vi "Post-Post-Build Action.vi"() -> ()   [LabVIEW 2020]
uses:
  <vilib>/JKI/VIPM API/command-line/support/Version Info Cluster_vipm_api.ctl
  <vilib>/Utility/miscctls.llb/LVMapReplaceAction.ctl
  <vilib>/Utility/traverseref.llb/TRef TravTarget.ctl
  cd8b867b-32d4-4915-be8a-6b797f053483.vi
  2e8c776f-19e2-48a1-b577-1ff0846f967f.vi
  383cdb5e-1483-4389-8633-9a82e05b406f.vi
  da8bf82a-4c59-4cf2-9509-83ebec40744a.vi
  <vilib>/Utility/traverseref.llb/VI Scripting - Traverse.lvlib
  <vilib>/JKI/VIPM API/VIPM API_vipm_api.lvlib
panel:
  out "File":path
  out "Action":string
  in  "Folder Path":path caption="Folder Path (Empty: Source Distrubution Built Folder)"
  # "Run this after the source distribution build and outside of the main project to avoid crashes/cross linking to VI.lib"
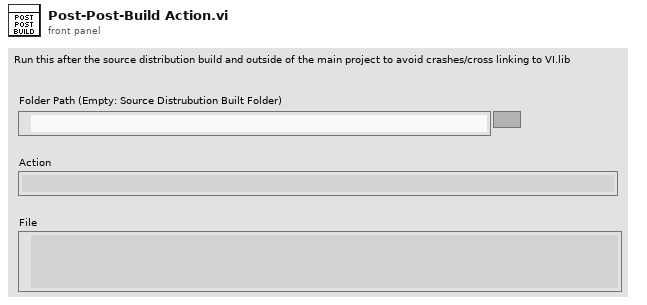
[diagram p1: front panel]
types:
  T1 = typedef "VIPM API_vipm_api.lvlib/Version Info Cluster_vipm_api.ctl" = cluster{"major":u32, "minor":u32, "patch":u32, "build":u32}
  T2 = cluster{"Vims":map{path, path[]}, "Src Files":path[]}
  T3 = cluster{"Source Distribution":path, "vi.lib Binary Source Dir":path, "Binary Source Dir":path}
  T4 = enum16{"Compute Paths", "Scan for .vims", "Inline .vims", "Delete .vims from Libs & Disk", "Rewildcard Paths before zip", "Zip", "Copy Binaries to vi.lib"}
  T5 = enum16{"Compute Paths", "Scan for .vims", "Inline .vims", "Delete .vims from Libs & Disk", "Rewildcard Paths before zip", "Zip", "Copy Binaries to vi.lib"}[]
  T6 = typedef "LVMapReplaceAction.ctl" = enum32{"Modify Entry only if found", "Add or Modify Entry", "Delete Entry"}
  T7 = typedef "TRef TravTarget.ctl" = enum16{"FP", "BD", "Other"}
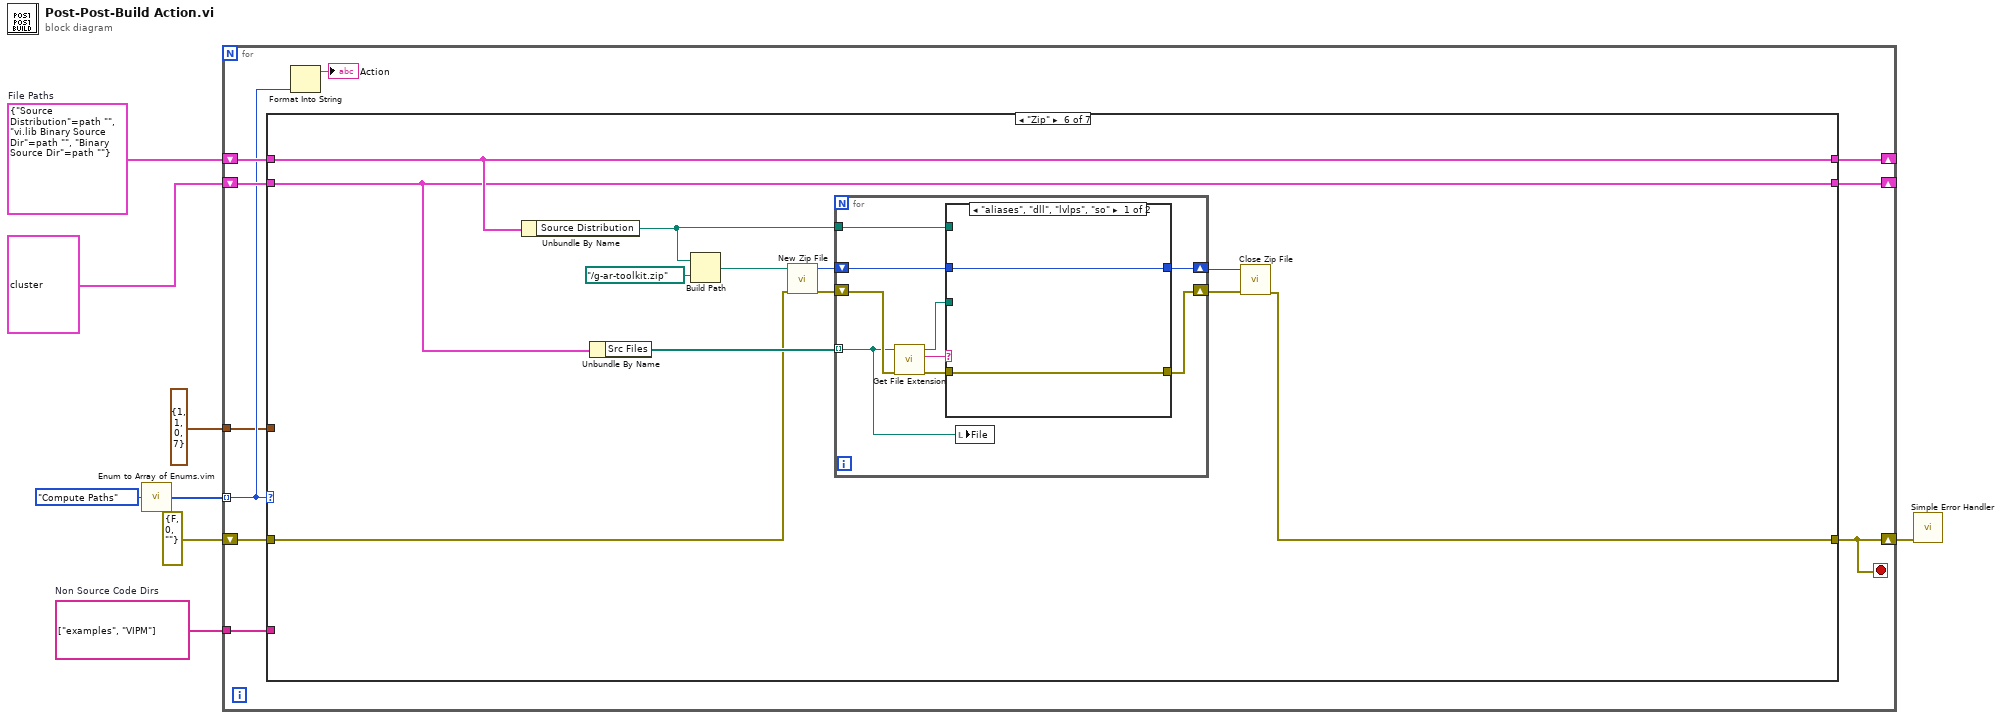
[diagram p0: block diagram]
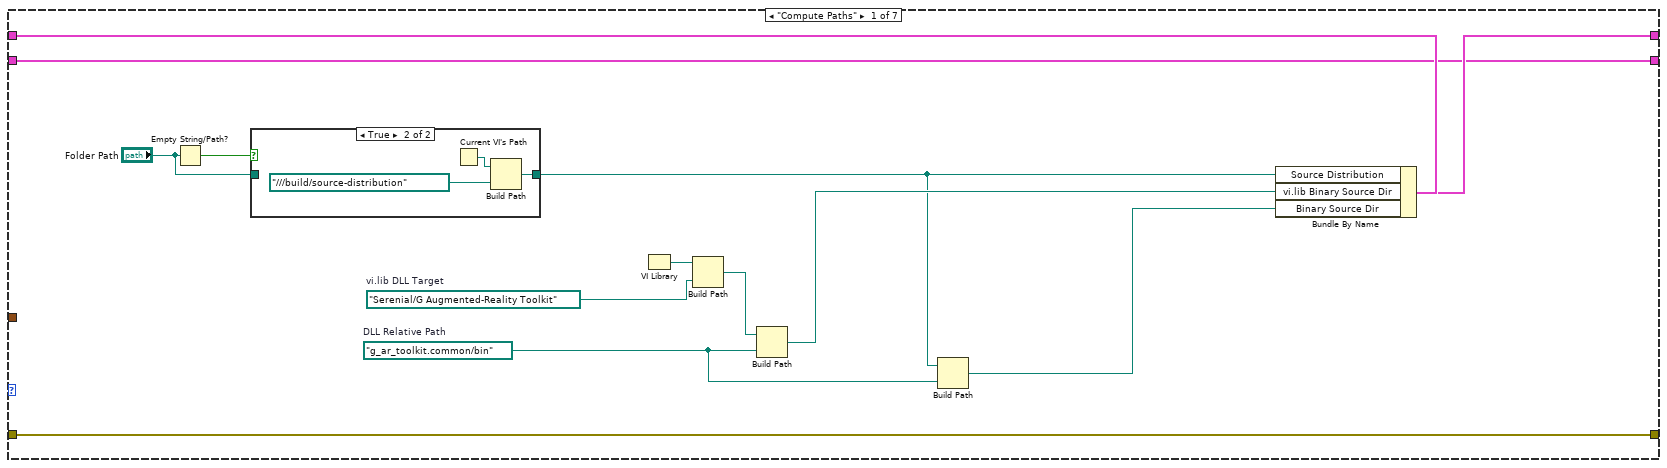
[diagram p2: hidden frame]
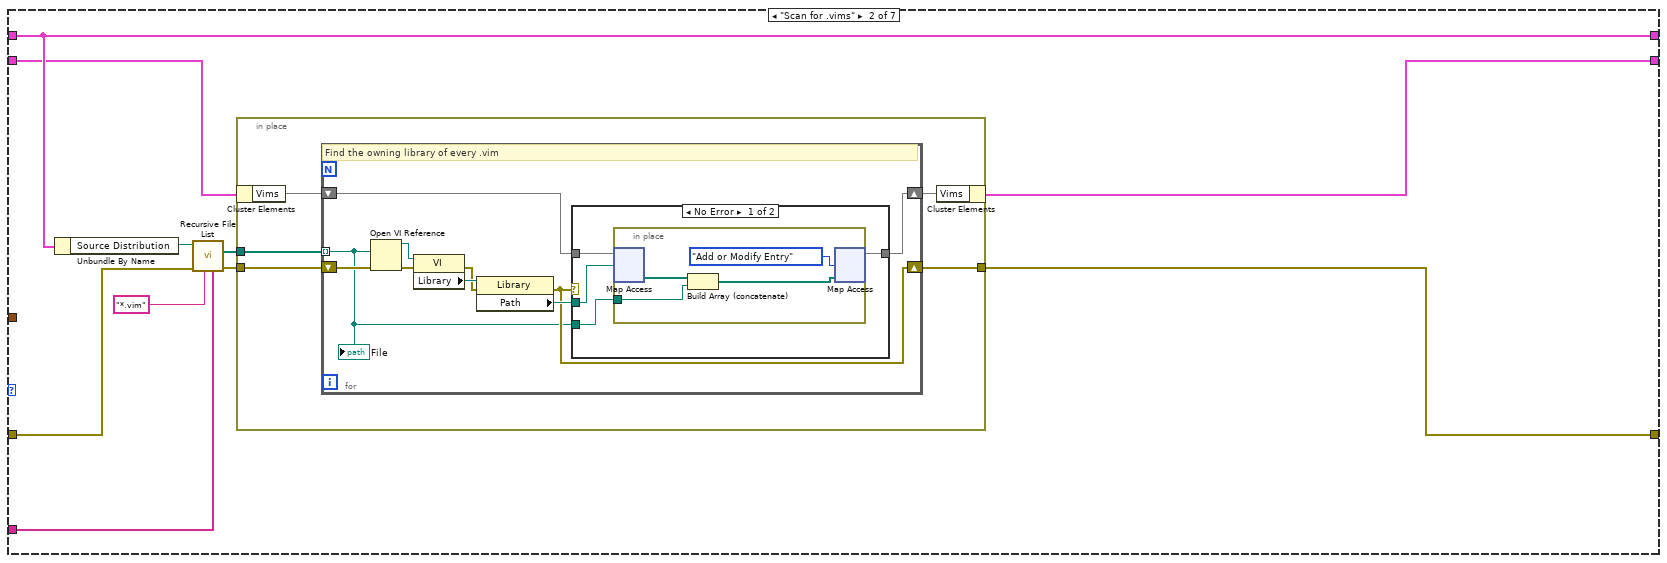
[diagram p4: hidden frame]
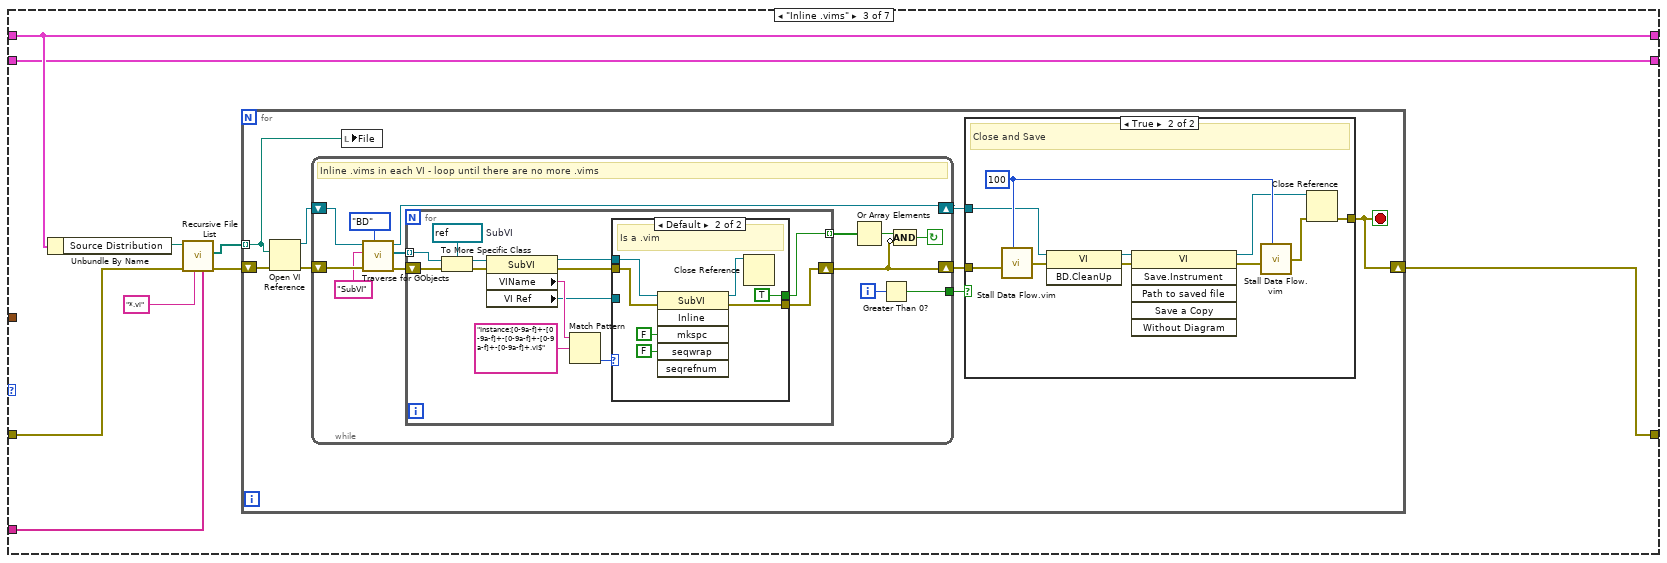
[diagram p6: hidden frame]
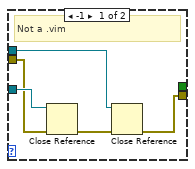
[diagram p7: hidden frame]
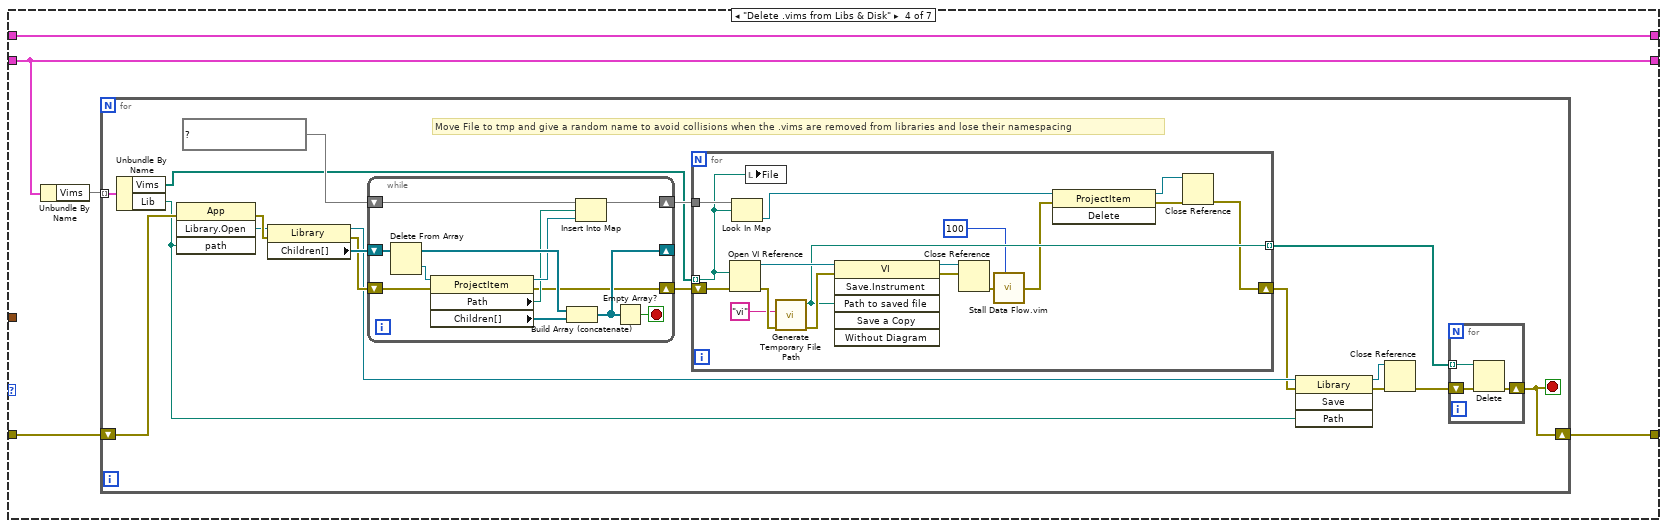
[diagram p9: hidden frame]
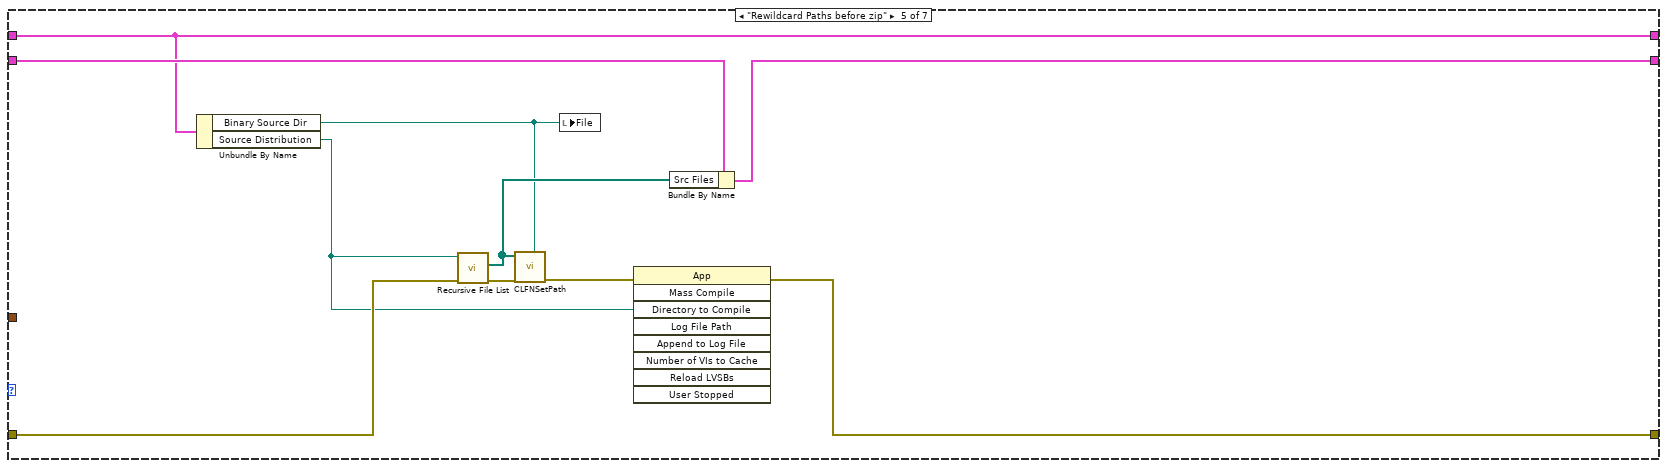
[diagram p10: hidden frame]
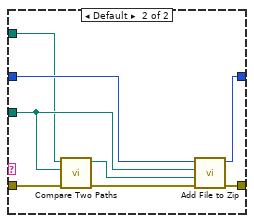
[diagram p11: hidden frame]
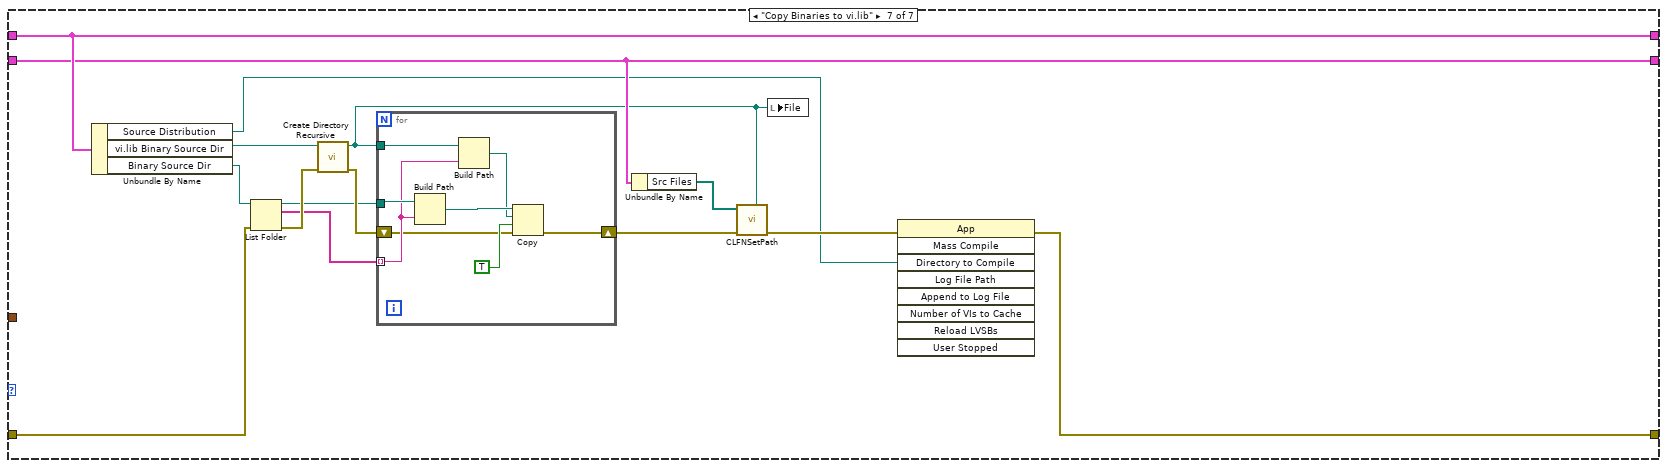
[diagram p12: hidden frame]
diagram:
  w4 = string[] ["examples", "VIPM"]  # Non Source Code Dirs
  w8 = T3 {"Source Distribution"=path "", "vi.lib Binary Source Dir"=path "", "Binary Source Dir"=path ""}  # File Paths
  n1 = call "Enum to Array of Enums.vim"("enum"=T4."Compute Paths") -> ("array of enums"=w6:T5)
  n2 = for {
    shift-right: [w17] -> _
    shift-left: w8 -> [w18]
    tunnel: w6 -> [w12] mode=indexing
    shift-right: [w10] -> w2
    shift-left: errorcluster {"status"=FALSE, "code"=0, "source"=""} ("error constant") -> [w16]
    tunnel: w4 -> [w15]
    shift-right: [w13] -> _
    shift-left: T2 {"Vims"={}, "Src Files"=[]} -> [w14]
    tunnel: T1 {"major"=1, "minor"=1, "patch"=0, "build"=7} ("Package Version") -> [w9]
    stop <- w10 stop-if-true
    n3 = case shown="\"Zip\"" w12 {
      tunnel: w18 -> [w29 w41 w76 w142 w201 w213 w248]
      tunnel: [w28 w41 w76 w142 w201 w213 w248] -> w17
      tunnel: w16 -> [w26 w40 w75 w141 w199 w208 w243]
      tunnel: w15 -> [_ w39 w74 _ _ _ _]
      tunnel: w14 -> [w27 w38 w71 w139 w202 w210 w239]
      tunnel: [w27 w37 w71 w139 w196 w210 w239] -> w13
      tunnel: [w26 w36 w73 w138 w197 w204 w236] -> w10
      tunnel: w9 -> [_ _ _ _ _ _ _]
      frame "Compute Paths" {
        w24 = path "Serenial/G Augmented-Reality Toolkit"  # vi.lib DLL Target
        w20 = path "g_ar_toolkit.common/bin"  # DLL Relative Path
        n4 = Empty String/Path?(string/path="Folder Path") -> (empty?=w31:bool)
        n5 = case shown="True" w31 {
          tunnel: [w32 w33] -> w21
          tunnel: "Folder Path" -> [w32 _]
          frame False {
          }
          frame True {
            n6 = Current VI's Path() -> (path=w35:path)
            n7 = Build Path(base path=w35, name or relative path=path "../../../build/source-distribution") -> (appended path=w33:path)
          }
        }
        n8 = VI Library() -> (path=w25:path)
        n9 = Build Path(base path=w25, name or relative path=w24) -> (appended path=w23:path)
        n10 = Build Path(base path=w23, name or relative path=w20) -> (appended path=w22:path)
        n11 = Build Path(base path=w21, name or relative path=w20) -> (appended path=w19:path)
        n12 = Bundle By Name(cluster=w29, "Source Distribution"=w21, "vi.lib Binary Source Dir"=w22, "Binary Source Dir"=w19) -> (w28:T3)
      }
      frame "Scan for .vims" {
        n13 = Unbundle By Name(w41) -> ("Source Distribution"=w42:path)
        n14 = call <vilib>:"Recursive File List.vi"("Folders to Exclude"=w39, "pattern"="*.vim", "error in (no error)"=w40, "Folder Path"=w42) -> ("error out"=w43:errorcluster, "All Files in Dir"=w44:path[])  [unwired: 3 in, 3 out]
        n15 = in-place {
          in-place-border: w44 -> [w50]
          in-place-border: w43 -> [w49]
          in-place-border: [w46] -> w36
          n16 = in-place-cluster #1(w38) -> ("Vims"=w48:map{path, path[]})
          n17 = for {
            tunnel: w50 -> [w51] mode=indexing
            shift-right: [w57] -> w47
            shift-left: w48 -> [w56]
            shift-right: [w52] -> w46
            shift-left: w49 -> [w60]
            # "Find the owning library of every .vim"
            n18 = Open VI Reference(vi path=w51, error in (no error)=w60) -> (vi reference=w59:refnum<vi>, error out=w58:errorcluster)  [unwired: 4 in]
            n19 = property class="VI"(reference=w59, error in=w58) -> (error out=w54:errorcluster, "Library"=w55:refnum<vi>)  [unwired: 1 out]
            n20 = property class="Library"(reference=w55, error in=w54) -> (error out=w52:errorcluster, "Path"=w53:path)  [unwired: 1 out]
            n21 = case shown="No Error" w52 {
              tunnel: [w64 w69] -> w57
              tunnel: w56 -> [w63 w69]
              tunnel: w53 -> [w62 _]
              tunnel: w51 -> [w61 _]
              frame No Error {
                n22 = in-place {
                  in-place-border: w61 -> [w66]
                  n23 = in-place-map #2(w63, w62) -> (w68:path[])  [unwired: 1 in, 1 out]
                  n24 = Build Array (concatenate)(w68, w66) -> (w65:path[])
                  n25 = in-place-map #2(w65, LVMapReplaceAction."Add or Modify Entry" ("action")) -> (w64:map{path, path[]})  [unwired: 2 out]
                }
              }
              frame Error {
              }
            }
            "File" <- w51
          }
          n26 = in-place-cluster #1("Vims"=w47) -> (w37:T2)
        }
      }
      frame "Inline .vims" {
        n27 = Unbundle By Name(w76) -> ("Source Distribution"=w77:path)
        n28 = call <vilib>:"Recursive File List.vi"("Folders to Exclude"=w74, "pattern"="*.vi", "error in (no error)"=w75, "Folder Path"=w77) -> ("error out"=w72:errorcluster, "All Files in Dir"=w70:path[])  [unwired: 3 in, 3 out]
        n29 = for {
          shift-right: [w81] -> w73
          shift-left: w72 -> [w84]
          tunnel: w70 -> [w79] mode=indexing
          stop <- w81 stop-if-true
          n30 = Open VI Reference(vi path=w79, error in (no error)=w84) -> (vi reference=w85:refnum<vi>, error out=w80:errorcluster)  [unwired: 4 in]
          n31 = while {
            shift-right: [w97] -> w82
            shift-left: w85 -> [w98]
            shift-right: [w87] -> w86
            shift-left: w80 -> [w96]
            tunnel: [w90] -> w83
            i -> [w91]
            stop <- w88 continue-if-true
            # "Inline .vims in each VI - loop until there are no more .vims"
            n32 = call <vilib>:"Traverse for GObjects.vi"("Traverse Target"=TRef_TravTarget."BD", "error in (no error)"=w96, "Class Name"="SubVI", "VI Refnum"=w98) -> ("error out"=w95:errorcluster, "References"=w93:refnum<vi>[], "dup VI Refnum"=w97:refnum<vi>)  [unwired: 4 in, 1 out]
            n33 = for {
              shift-right: [w100] -> w87
              shift-left: w95 -> [w112]
              tunnel: w93 -> [w111] mode=indexing
              tunnel: [w106] -> w99 mode=indexing
              w110 = refnum<vi> refnum  # SubVI
              n34 = To More Specific Class(target class=w110, reference=w111, error in=w112) -> (specific class reference=w109:refnum<vi>, error out=w108:errorcluster)
              n35 = property class="SubVI"(reference=w109, error in=w108) -> (reference out=w102:refnum<vi>, error out=w105:errorcluster, "VIName"=w107:string, "VI Ref"=w103:refnum<vi>)
              n36 = Match Pattern(string=w107, regular expression="Instance:[0-9a-f]+-[0-9a-f]+-[0-9a-f]+-[0-9a-f]+-[0-9a-f]+.vi$") -> (offset past match=w104:i32)  [unwired: 1 in, 3 out]
              n37 = case shown="Default" w104 {
                tunnel: [w117 w124] -> w100
                tunnel: w103 -> [w115 _]
                tunnel: [_ TRUE] -> w106
                tunnel: w105 -> [w113 w119]
                tunnel: w102 -> [w116 w122]
                frame -1 {
                  # "Not a .vim"
                  n38 = Close Reference(reference=w115, error in (no error)=w113) -> (error out=w114:errorcluster)
                  n39 = Close Reference(reference=w116, error in (no error)=w114) -> (error out=w117:errorcluster)
                }
                frame Default {
                  # "Is a .vim"
                  n40 = invoke class="SubVI" method="Inline"(reference=w122, error in=w119, "mkspc"=FALSE ("Make Space in Block Diagram"), "seqwrap"=FALSE ("Wrap in Sequence")) -> (reference out=w118:refnum<vi>, error out=w124:errorcluster)  [unwired: 2 in, 4 out]
                  n41 = Close Reference(reference=w118) -> ()  [unwired: 1 in, 1 out]
                }
              }
            }
            n42 = Or Array Elements(Boolean array=w99) -> (logical OR=w92:bool)
            n43 = Greater Than 0?(x=w91) -> (x > 0?=w90:bool)
            n44 = Compound Arithmetic op=AND(w92, invert w87) -> (w88:bool)
          }
          n45 = local write "File"(w79) -> ()
          n46 = case shown="True" w83 {
            tunnel: w82 -> [w125 w129]
            tunnel: w86 -> [w127 w137]
            tunnel: [w126 w128] -> w81
            frame False {
              # "No Updates"
              n47 = Close Reference(reference=w125, error in (no error)=w127) -> (error out=w126:errorcluster)
            }
            frame True {
              w131 = u32 100 ("milliseconds to wait")
              # "Close and Save"
              n48 = call "Stall Data Flow.vim"("value in"=w137, "milliseconds to wait"=w131) -> ("value out"=w133:errorcluster)  [unwired: 1 out]
              n49 = invoke class="VI" method="BD.CleanUp"(reference=w129, error in=w133) -> (reference out=w136:refnum<vi>, error out=w135:errorcluster)  [unwired: 1 in, 1 out]
              n50 = invoke class="VI" method="Save.Instrument"(reference=w136, error in=w135) -> (reference out=w130:refnum<vi>, error out=w134:errorcluster)  [unwired: 4 in, 4 out]
              n51 = call "Stall Data Flow.vim"("value in"=w134, "milliseconds to wait"=w131) -> ("value out"=w132:errorcluster)  [unwired: 1 out]
              n52 = Close Reference(reference=w130, error in (no error)=w132) -> (error out=w128:errorcluster)
            }
          }
        }
      }
      frame "Delete .vims from Libs & Disk" {
        n53 = Unbundle By Name(w139) -> ("Vims"=w140:map{path, path[]})
        n54 = for {
          shift-right: [w143] -> w138
          shift-left: w141 -> [w159]
          tunnel: w140 -> [w160] mode=indexing
          stop <- w143 stop-if-true
          # "Move File to tmp and give a random name to avoid collisions when the .vims are removed from libraries and lose their namespacing"
          n55 = Unbundle By Name(w160) -> ("Vims"=w155:path[], "Lib"=w149:path)
          n56 = invoke class="App" method="Library.Open"(error in=w159, "path"=w149) -> (error out=w154:errorcluster, "Open Library"=w148:refnum<vi>)  [unwired: 2 in, 2 out]
          n57 = property class="Library"(reference=w148, error in=w154) -> (reference out=w151:refnum<vi>, error out=w153:errorcluster, "Children[]"=w158:refnum<vi>[])
          n58 = while {
            shift-right: [w169] -> _
            shift-left: w158 -> [w175]
            shift-right: [w171] -> w156
            shift-left: map{path, refnum<vi>} {} ("Size: 0") -> [w170]
            shift-right: [w164] -> w152
            shift-left: w153 -> [w167]
            stop <- w168 stop-if-true
            n59 = Delete From Array(array=w175) -> (deleted portion=w174:refnum<vi>, array with subset deleted=w173:refnum<vi>[])  [unwired: 2 in]
            n60 = property class="ProjectItem"(reference=w174, error in=w167) -> (reference out=w172:refnum<vi>, error out=w164:errorcluster, "Path"=w165:path, "Children[]"=w166:refnum<vi>[])
            n61 = Build Array (concatenate)(w173, w166) -> (w169:refnum<vi>[])
            n62 = Insert Into Map(map in=w170, key=w165, value=w172) -> (map out=w171:map{path, refnum<vi>})  [unwired: 2 out]
            n63 = Empty Array?(array=w169) -> (empty?=w168:bool)
          }
          n64 = for {
            shift-right: [w176] -> w150
            shift-left: w152 -> [w191]
            tunnel: w155 -> [w183] mode=indexing
            tunnel: [w179] -> w145 mode=indexing
            tunnel: w156 -> [w192]
            n65 = Open VI Reference(vi path=w183, error in (no error)=w191) -> (vi reference=w188:refnum<vi>, error out=w182:errorcluster)  [unwired: 4 in]
            n66 = Look In Map(map=w192, key=w183) -> (value=w189:refnum<vi>)  [unwired: 1 in, 1 out]
            n67 = local write "File"(w183) -> ()
            n68 = call <vilib>:"Generate Temporary File Path.vi"("error in (no error)"=w182, "Temporary File Extension (tmp)"="vi") -> ("error out"=w180:errorcluster, "Unique Temporary File Path"=w179:path)  [unwired: 8 in]
            n69 = invoke class="VI" method="Save.Instrument"(reference=w188, error in=w180, "Path to saved file"=w179) -> (reference out=w186:refnum<vi>, error out=w190:errorcluster)  [unwired: 3 in, 4 out]
            n70 = Close Reference(reference=w186, error in (no error)=w190) -> (error out=w187:errorcluster)
            n71 = call "Stall Data Flow.vim"("value in"=w187, "milliseconds to wait"=u32 100) -> ("value out"=w177:errorcluster)  [unwired: 1 out]
            n72 = invoke class="ProjectItem" method="Delete"(reference=w189, error in=w177) -> (reference out=w184:refnum<vi>, error out=w185:errorcluster)  [unwired: 1 in, 1 out]
            n73 = Close Reference(reference=w184, error in (no error)=w185) -> (error out=w176:errorcluster)
          }
          n74 = invoke class="Library" method="Save"(reference=w151, error in=w150, "Path"=w149) -> (reference out=w146:refnum<vi>, error out=w147:errorcluster)  [unwired: 1 in, 2 out]
          n75 = Close Reference(reference=w146, error in (no error)=w147) -> (error out=w144:errorcluster)
          n76 = for {
            tunnel: w145 -> [w161] mode=indexing
            shift-right: [w162] -> w143
            shift-left: w144 -> [w163]
            n77 = Delete(path (use dialog)=w161, error in=w163) -> (error out=w162:errorcluster)  [unwired: 3 in, 2 out]
          }
        }
      }
      frame "Rewildcard Paths before zip" {
        n78 = Unbundle By Name(w201) -> ("Binary Source Dir"=w193:path, "Source Distribution"=w194:path)
        n79 = call <vilib>:"Recursive File List.vi"("error in (no error)"=w199, "Folder Path"=w194) -> ("error out"=w200:errorcluster, "All Files in Dir"=w195:path[])  [unwired: 5 in, 3 out]
        n80 = call "CLFNSetPath.vi"("New Root Path"=w193, "error in (no error)"=w200, "Files"=w195) -> ("error out"=w198:errorcluster)  [unwired: 8 in]
        n81 = local write "File"(w193) -> ()
        n82 = invoke class="App" method="Mass Compile"(error in=w198, "Directory to Compile"=w194) -> (error out=w197:errorcluster)  [unwired: 7 in, 8 out]
        n83 = Bundle By Name(cluster=w202, "Src Files"=w195) -> (w196:T2)
      }
      frame "Zip" {
        n84 = Unbundle By Name(w213) -> ("Source Distribution"=w203:path)
        n85 = Unbundle By Name(w210) -> ("Src Files"=w209:path[])
        n86 = Build Path(base path=w203, name or relative path=path "../g-ar-toolkit.zip") -> (appended path=w211:path)
        n87 = call <vilib>:"New Zip File.vi"("error in (no error)"=w208, "target"=w211) -> ("error out"=w214:errorcluster, "zip file out"=w207:i64)  [unwired: 3 in, 1 out]
        n88 = for {
          shift-right: [w221] -> w205
          shift-left: w207 -> [w223]
          shift-right: [w222] -> w206
          shift-left: w214 -> [w220]
          tunnel: w209 -> [w215] mode=indexing
          tunnel: w203 -> [w216]
          n89 = call <vilib>:"Get File Extension.vi"("error in (no error)"=w220, "file"=w215) -> ("error out"=w219:errorcluster, "lowercase file extension"=w217:string, "dup file"=w218:path)  [unwired: 5 in, 2 out]
          n90 = case shown="\"aliases\", \"dll\", \"lvlps\", \"so\"" w217 {
            tunnel: w223 -> [w224 w232]
            tunnel: [w225 w230] -> w222
            tunnel: [w224 w229] -> w221
            tunnel: w218 -> [_ w227]
            tunnel: w219 -> [w225 w228]
            tunnel: w216 -> [_ w226]
            frame "aliases", "dll", "lvlps", "so" {
            }
            frame Default {
              n91 = call <vilib>:"Compare Two Paths.vi"("error in (no error)"=w228, "Path 2"=w227, "Path 1"=w226) -> ("error out"=w231:errorcluster, "Relative Path from 1 to 2"=w233:path)  [unwired: 5 in, 2 out]
              n92 = call <vilib>:"Add File to Zip.vi"("error in (no error)"=w231, "destination path in zip"=w233, "source file path"=w227, "zip file in"=w232) -> ("error out"=w230:errorcluster, "zip file out"=w229:i64)  [unwired: 6 in]
            }
          }
          n93 = local write "File"(w215) -> ()
        }
        n94 = call <vilib>:"Close Zip File.vi"("error in (no error)"=w206, "zip file in"=w205) -> ("error out"=w204:errorcluster)  [unwired: 5 in]
      }
      frame "Copy Binaries to vi.lib" {
        n95 = Unbundle By Name(w248) -> ("Source Distribution"=w235:path, "vi.lib Binary Source Dir"=w246:path, "Binary Source Dir"=w247:path)
        n96 = List Folder(path=w247, error in=w243) -> (path out=w242:path, filenames=w241:string[], error out=w245:errorcluster)  [unwired: 2 in, 1 out]
        n97 = call <vilib>:"Create Directory Recursive.vi"("error in (no error)"=w245, "directory"=w246) -> ("error out"=w244:errorcluster, "directory copy"=w234:path)  [unwired: 3 in, 1 out]
        n98 = for {
          tunnel: w242 -> [w256]
          tunnel: w241 -> [w253] mode=indexing
          tunnel: w234 -> [w254]
          shift-right: [w249] -> w240
          shift-left: w244 -> [w250]
          n99 = Build Path(base path=w256, name or relative path=w253) -> (appended path=w255:path)
          n100 = Build Path(base path=w254, name or relative path=w253) -> (appended path=w252:path)
          n101 = Copy(8:w250, 9:TRUE ("overwrite (F)"), 10:w252, 11:w255) -> (0:w249:errorcluster)  [unwired: 1 in, 2 out]
        }
        n102 = Unbundle By Name(w239) -> ("Src Files"=w238:path[])
        n103 = call "CLFNSetPath.vi"("New Root Path"=w234, "error in (no error)"=w240, "Files"=w238) -> ("error out"=w237:errorcluster)  [unwired: 8 in]
        n104 = local write "File"(w234) -> ()
        n105 = invoke class="App" method="Mass Compile"(error in=w237, "Directory to Compile"=w235) -> (error out=w236:errorcluster)  [unwired: 7 in, 8 out]
      }
    }
    n106 = Format Into String(w12) -> (resulting string=→"Action":string)  [unwired: 3 in, 1 out]
  }
  n107 = call <vilib>:"Simple Error Handler.vi"("error in (no error)"=w2) -> ()  [unwired: 4 in, 5 out]
